vi "Stanford Research 830 Acquire Measurement - All Parameters.vi"() -> ()   [LabVIEW 2017]
doc: "This example shows how to configure the instrument to read all the parameters available."
uses:
  <instrlib>/Stanford Research 830/Public/Data/Read (All Parameters).vi
  <instrlib>/Stanford Research 830/Stanford Research 830.lvlib
panel:
  in  "Internal Reference Frequency (1000 Hz)":dbl=1000.0
  in  "Sine Output Amplitude (1 V)":dbl=1.0
  out "Parameter Values":T1
  in  "Sensitivity (26: 1 V/uA)":i16(ring)=26 items=["Auto Gain"=-1, "2 nV/fA"=0, "5 nV/fA"=1, "10 nV/fA"=2, "20 nV/fA"=3, "50 nV/fA"=4, "100 nV/fA"=5, "200 nV/fA"=6, "500 nV/fA"=7, "1 uV/pA"=8, "2 uV/pA"=9, "5 uV/pA"=10, "10 uV/pA"=11, "20 uV/pA"=12, "50 uV/pA"=13, "100 uV/pA"=14, "200 uV/pA"=15, "500 uV/pA"=16, "1 mV/nA"=17, "2 mV/nA"=18, "5 mV/nA"=19, "10 mV/nA"=20, "20 mV/nA"=21, "50 mV/nA"=22, "100 mV/nA"=23, "200 mV/nA"=24, "500 mV/mA"=25, "1 V/uA"=26]
  in  "Dynamic Reserve (2: Low Noise)":i16(ring)=2 items=["High Reserve"=0, "Normal"=1, "Low Noise"=2, "Auto Reserve"=-1]
  in  "Reference Source (1: Internal)":u16(ring)=1 items=["External", "Internal"]
  in  "Input Coupling (0: AC)":u16(ring) items=["AC", "DC"]
  in  "Input Connection (0: Single-Ended Voltage)":u16(ring) items=["Single-Ended Voltage", "Differential Voltage", "1 MOhm Current Gain", "100 MOhm Current Gain"]
  in  "VISA":refnum<visa-resource-name>
  # "Input Signal"
  # "Reference"
  # "Sensitivity and Reserve"
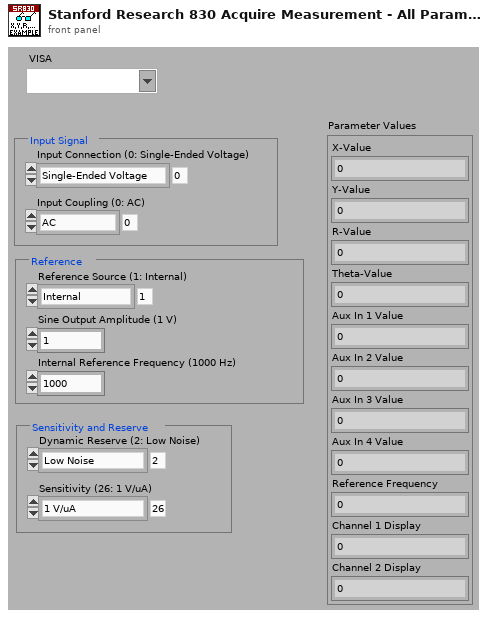
[diagram p1: front panel]
types:
  T1 = cluster{"X-Value":dbl, "Y-Value":dbl, "R-Value":dbl, "Theta-Value":dbl, "Aux In 1 Value":dbl, "Aux In 2 Value":dbl, "Aux In 3 Value":dbl, "Aux In 4 Value":dbl, "Reference Frequency":dbl, "Channel 1 Display":dbl, "Channel 2 Display":dbl}
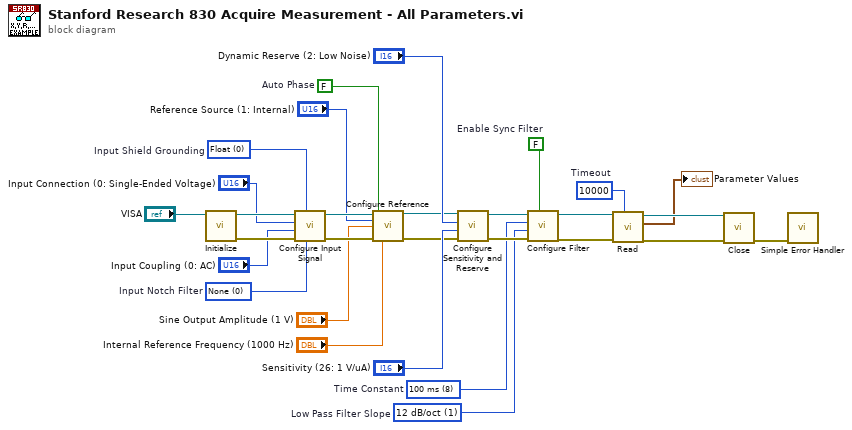
[diagram p0: block diagram]
diagram:
  w1 = FALSE  # Enable Sync Filter
  w2 = u16 1 items=["6 dB/oct", "12 dB/oct", "18 db/oct", "24 dB/oct"]  # Low Pass Filter Slope
  w3 = u16 8 items=["10 us", "30 us", "100 us", "300 us", "1 ms", "3 ms", "10 ms", "30 ms", "100 ms", "300 ms", "1 s", "3 s", "10 s", "30 s", "100 s", "300 s", "1 ks", "3 ks", "10 ks", "30 ks"]  # Time Constant
  w10 = u32 10000  # Timeout
  w19 = FALSE  # Auto Phase
  w20 = u16 0 items=["None", "Line Notch", "2x Line Notch", "Both Notch Filters"]  # Input Notch Filter
  w21 = u16 0 items=["Float", "Ground"]  # Input Shield Grounding
  n1 = call <instrlib>:"Initialize.vi"("VISA resource name"="VISA") -> ("error out"=w28:errorcluster, "VISA resource name out"=w27:refnum<visa-resource-name>)  [unwired: 9 in]
  n2 = call <instrlib>:"Configure Input Signal.vi"("Input Notch Filter (0: None)"=w20, "Input Shield Grounding (0: Float)"=w21, "error in (no error)"=w28, "Input Coupling (0: AC)"="Input Coupling (0: AC)", "Input Connection (0: Single-Ended Voltage)"="Input Connection (0: Single-Ended Voltage)", "VISA resource name"=w27) -> ("error out"=w25:errorcluster, "VISA resource name out"=w26:refnum<visa-resource-name>)  [unwired: 4 in]
  n3 = call <instrlib>:"Configure Reference.vi"("VISA resource name"=w26, "Auto Phase (T: Enabled)"=w19, "Reference Source (1: Internal)"="Reference Source (1: Internal)", "Sine Output Amplitude (1 V)"="Sine Output Amplitude (1 V)", "error in (no error)"=w25, "Internal Reference Frequency (1000 Hz)"="Internal Reference Frequency (1000 Hz)") -> ("VISA resource name out"=w14:refnum<visa-resource-name>, "error out"=w13:errorcluster)  [unwired: 8 in]
  n4 = call <instrlib>:"Configure Sensitivity and Reserve.vi"("error in (no error)"=w13, "Sensitivity (-1: Auto gain)"="Sensitivity (26: 1 V/uA)", "Dynamic Reserve (-1: Auto Reserve)"="Dynamic Reserve (2: Low Noise)", "VISA resource name"=w14) -> ("error out"=w6:errorcluster, "VISA resource name out"=w7:refnum<visa-resource-name>)  [unwired: 6 in]
  n5 = call <instrlib>:"Configure Filter.vi"("Enable Sync Filter (F: Disable)"=w1, "error in (no error)"=w6, "Low Pass Filter Slope (1: 12dB/oct)"=w2, "Time Constant (8: 100ms)"=w3, "VISA resource name"=w7) -> ("error out"=w4:errorcluster, "VISA resource name out"=w5:refnum<visa-resource-name>)  [unwired: 5 in]
  n6 = call-poly <instrlib>:"Read.vi"("Timeout (10000 ms)"=w10, "error in (no error)"=w4, "VISA resource name"=w5) -> ("error out"=w17:errorcluster, "Parameter Values"=→"Parameter Values":T1, "VISA resource name out"=w18:refnum<visa-resource-name>)  [unwired: 6 in]
  n7 = call <instrlib>:"Close.vi"("error in (no error)"=w17, "VISA resource name"=w18) -> ("error out"=w24:errorcluster)  [unwired: 9 in]
  n8 = call <vilib>:"Simple Error Handler.vi"("error in (no error)"=w24) -> ()  [unwired: 4 in, 5 out]
